vi "Experimento 1-1.vi"() -> ()   [LabVIEW 2010]
uses:
  <vilib>/express/express analysis/Spectral/XNode/ExpressSpectralMeasurementsBlockNode.xnode
  <vilib>/express/express analysis/Spectral/Block/exnSpectralBlock spectral measurements RMS poly.vi
  <vilib>/express/express analysis/Spectral/Block/exnSpectralBlock spectral measurements RMS DDT.vi
panel:
  out "Arquivo":string
  out "Frequncia (fase)":dynamicdata(graph)
  out "Frequncia (magnitude)":dynamicdata(graph)
  out "Tempo":dynamicdata(graph)
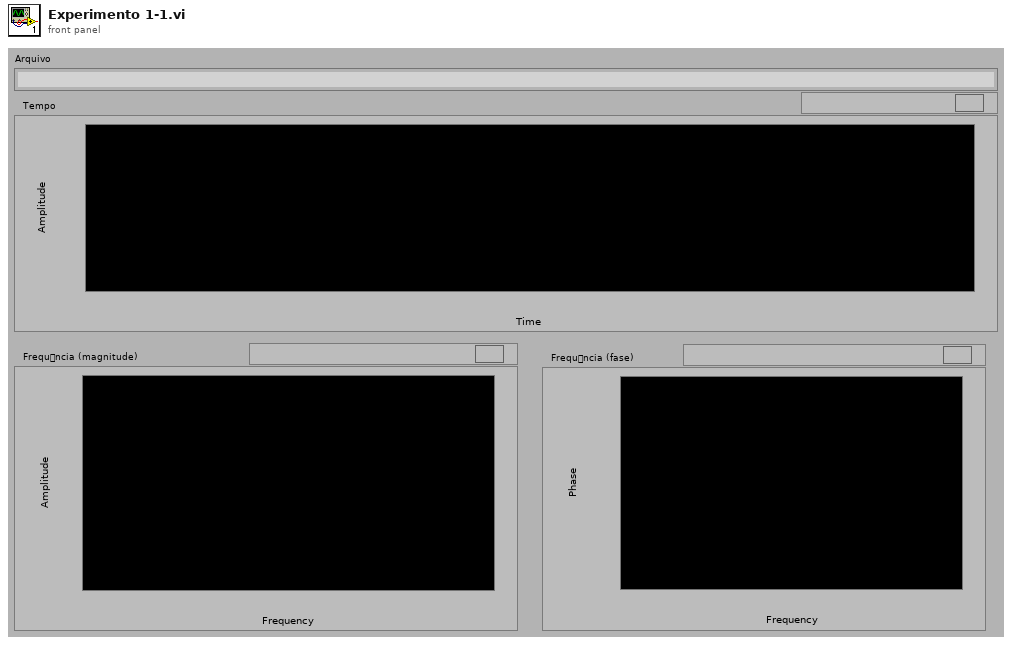
[diagram p1: front panel]
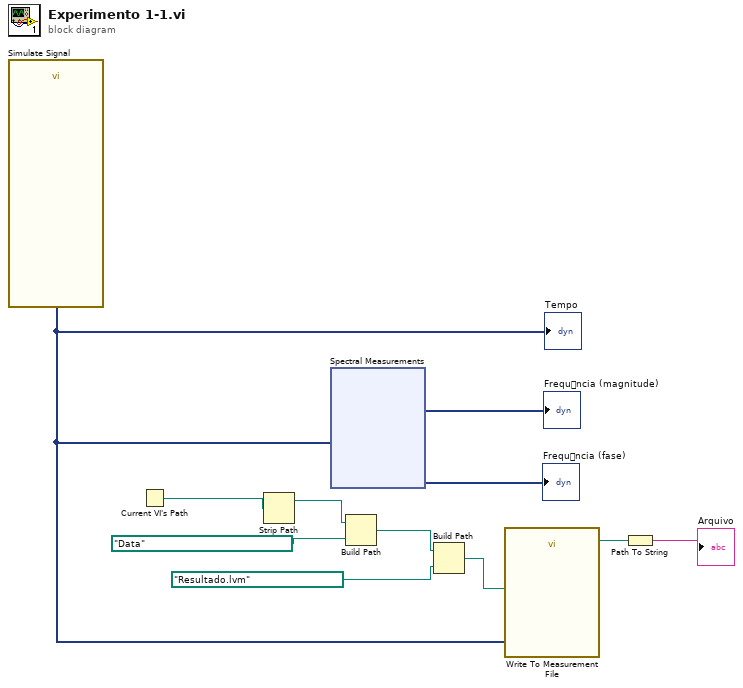
[diagram p0: block diagram]
diagram:
  n1 = call "Simulate Signal"() -> ("Sine with Uniform Noise"=w9:dynamicdata)  [unwired: 14 in, 1 out]
  "Tempo" <- w9
  n2 = Current VI's Path() -> (path=w6:path)
  n3 = Strip Path(path=w6) -> (stripped path=w7:path)  [unwired: 1 out]
  n4 = xnode "Spectral Measurements"("Signals"=w9) -> ("FFT - (RMS)"=→"Frequncia (magnitude)":dynamicdata, "Phase"=→"Frequncia (fase)":dynamicdata)  [unwired: 1 in, 1 out]
  n5 = Build Path(base path=w7, name or relative path=path "Data") -> (appended path=w3:path)
  n6 = Build Path(base path=w3, name or relative path=path "Resultado.lvm") -> (appended path=w1:path)
  n7 = call "Write To Measurement File"("Signals"=w9, "Filename"=w1) -> ("Filename Out"=w5:path)  [unwired: 15 in, 2 out]
  n8 = Path To String(path=w5) -> (string=→"Arquivo":string)
